vi "Substitute String.vi"(6 "delimeters":cluster{"start":string, "end":string}={"start"="{{", "end"="}}"}, 8 "error in (no error)":errorcluster, 9 "substitutions":map{string, string}(c390), 11 "input string":string) -> (0 "error out":errorcluster, 3 "output string":string)   [LabVIEW 2019]
doc: "<b>Description</b> This VI applies substitutions to the input string using the specified delimeters and substitution lookup table. \n\nFor example, the input string \"{{greeting}}, {{name}}\" would result in the output string \"Hello, World\" if the substituion dictionary contained the mappings {'greeting':'Hello', 'name':'World'}.\n\nThis VI will return an error if the input contains a substitution not found in the dictionary.\n\n\n\n<b>Inputs</b>\n<b>substitutions</b>: A dictoinary of substitutions to apply to the input string.\n<b>delimeters</b>: The start and end delimeters for the desired substitution pattern. Defaults to '{{' and '}}'.\n<b>input string</b>: A string potentially containing substituions.\n\n<b>Outputs</b>\n<b>error out</b>: This VI will return error -1967345147 if a substitution key is missing from the input dictionary.\n<b>output string</b>: A string with substitution keys replaced with values."
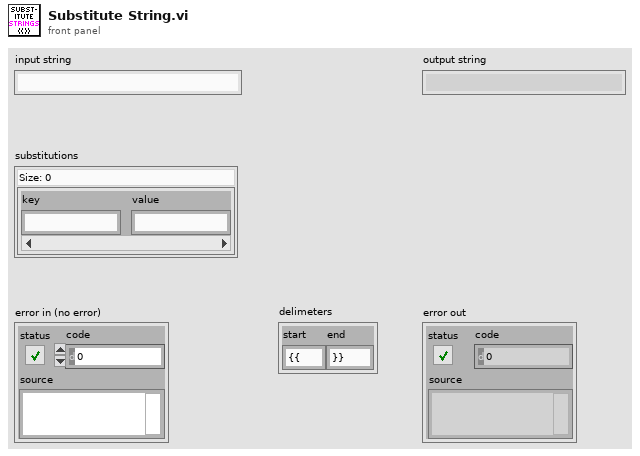
[diagram p1: front panel]
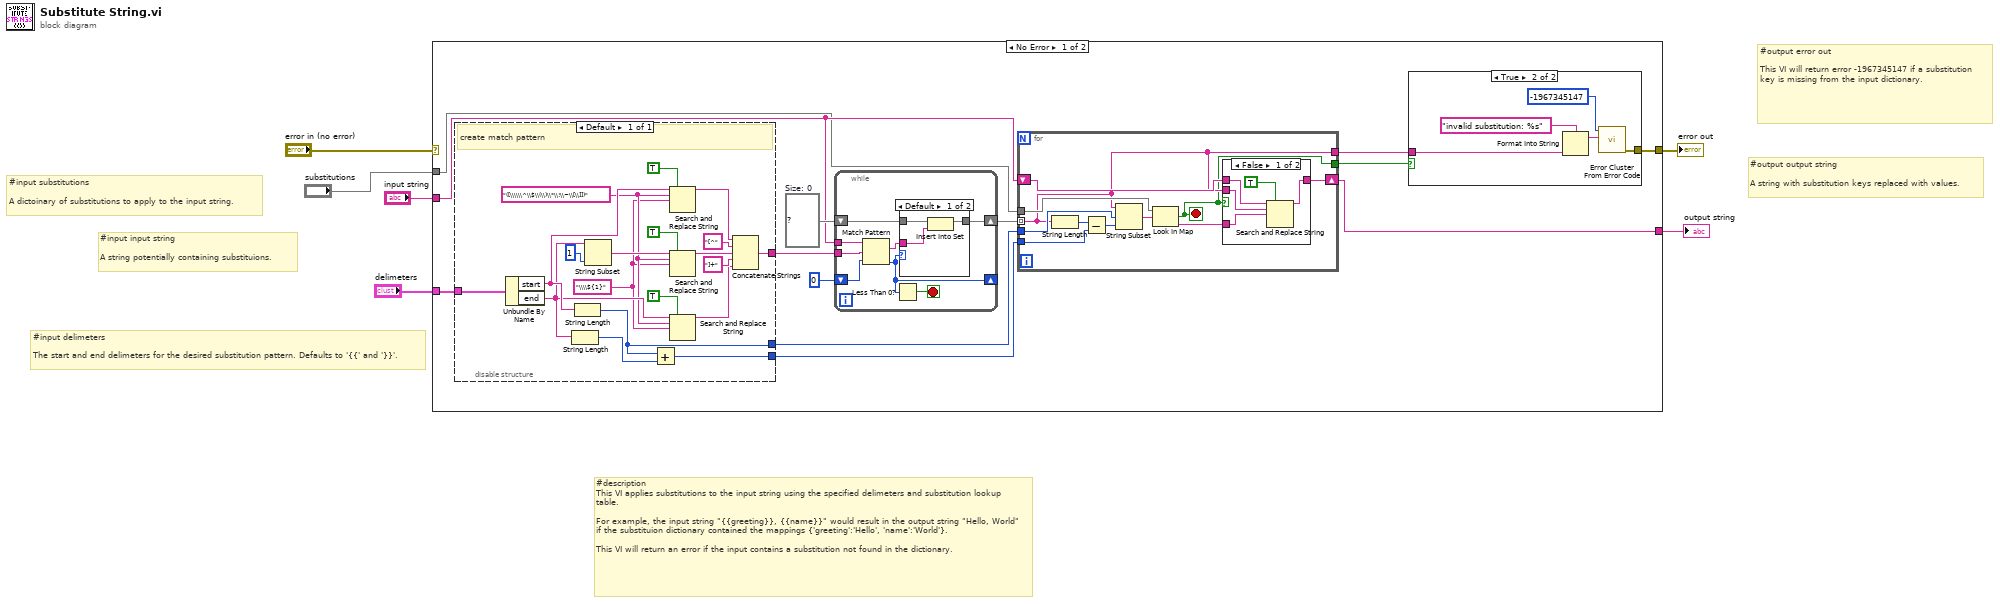
[diagram p0: block diagram]
diagram:
  # "#output error out\n\nThis VI will return error -1967345147 if a substitution key is missing from the input dictionary."
  # "#output output string\n\nA string with substitution keys replaced with values."
  # "#input substitutions\n\nA dictoinary of substitutions to apply to the input string."
  # "#input delimeters\n\nThe start and end delimeters for the desired substitution pattern. Defaults to '{{' and '}}'."
  # "#input input string\n\nA string potentially containing substituions."
  # "#description\nThis VI applies substitutions to the input string using the specified delimeters and substitution lookup table. \n\nFor example, the input string \"{{greeting}}, {{name}}\" would result in the output string \"Hello, World\" if the substituion dictionary contained the mappings {'greeting':'Hello', 'name':'World'}.\n\nThis VI will return an error if the input contains a substitution not found in the dictionary."
  n1 = case shown="No Error" "error in (no error)" {
    selector: "error in (no error)" -> [_ w73]
    tunnel: "delimeters" -> [w19 _]
    tunnel: "input string" -> [w15 _]
    tunnel: "substitutions" -> [w13 _]
    tunnel: [w8 w73] -> w2
    tunnel: [w7 _] -> w1
    frame No Error {
      w17 = set{string} {}  # Size: 0
      n2 = disable-structure shown="Default" {
        disable-tunnel: w19 -> [w60]
        disable-tunnel: [w57] -> w18
        disable-tunnel: [w54] -> w11
        disable-tunnel: [w53] -> w12
        frame Enabled {
          w46 = "\\\\${1}" ("replace string (\"\")")
          w47 = "([\\\\\\^\\$\\(\\)\\*\\!\\~\\[\\]])" ("search string")
          # "create match pattern"
          n3 = Unbundle By Name(w60) -> ("start"=w56:string, "end"=w52:string)
          n4 = String Length(string=w52) -> (length=w55:i32)
          n5 = String Length(string=w56) -> (length=w54:i32)
          n6 = String Subset(string=w52, length (rest)=1 ("length (rest)")) -> (substring=w48:string)  [unwired: 1 in]
          n7 = Add(x=w54, y=w55) -> (x+y=w53:i32)
          n8 = Search and Replace String(replace all?=TRUE ("replace all? (F)"), input string=w56, search string=w47, replace string=w46) -> (result string=w59:string)  [unwired: 4 in, 3 out]
          n9 = Search and Replace String(replace all?=TRUE ("replace all? (F)"), input string=w48, search string=w47, replace string=w46) -> (result string=w44:string)  [unwired: 4 in, 3 out]
          n10 = Search and Replace String(replace all?=TRUE ("replace all? (F)"), input string=w52, search string=w47, replace string=w46) -> (result string=w42:string)  [unwired: 4 in, 3 out]
          n11 = Concatenate Strings(w59, "[^" ("string"), w44, "]+" ("string"), w42) -> (w57:string)
        }
      }
      n12 = while {
        tunnel: w15 -> [w68]
        tunnel: w18 -> [w67]
        shift-right: [w63] -> w14
        shift-left: w17 -> [w64]
        shift-right: [w62] -> _
        shift-left: 0 ("offset past match") -> [w61]
        stop <- w66 stop-if-true
        n13 = Match Pattern(string=w68, regular expression=w67, offset (0)=w61) -> (match substring=w65:string, offset past match=w62:i32)  [unwired: 2 out]
        n14 = Less Than 0?(x=w62) -> (x < 0?=w66:bool)
        n15 = case shown="Default" w62 {
          tunnel: w65 -> [w69 _]
          tunnel: w64 -> [w71 w72]
          tunnel: [w70 w72] -> w63
          frame Default {
            n16 = Insert Into Set(10:w69, 11:w71) -> (3:w70:set{string})  [unwired: 1 out]
          }
          frame -1 {
          }
        }
      }
      n17 = for {
        shift-right: [w27] -> w7
        shift-left: w15 -> [w28]
        tunnel: w14 -> [w26] mode=indexing
        tunnel: w13 -> [w31]
        tunnel: w12 -> [w33]
        tunnel: w11 -> [w32]
        tunnel: [w25] -> w10
        tunnel: [w26] -> w9
        stop <- w25 stop-if-true
        n18 = String Length(string=w26) -> (length=w35:i32)
        n19 = Subtract(x=w35, y=w33) -> (x-y=w34:i32)
        n20 = String Subset(string=w26, offset (0)=w32, length (rest)=w34) -> (substring=w30:string)
        n21 = Look In Map(map=w31, key=w30) -> (key not found?=w25:bool, value=w29:string)  [unwired: 1 in]
        n22 = case shown="False" w25 {
          tunnel: w29 -> [w40 _]
          tunnel: w28 -> [w38 w41]
          tunnel: [w37 w41] -> w27
          tunnel: w26 -> [w36 _]
          frame False {
            n23 = Search and Replace String(replace all?=TRUE ("replace all? (F)"), input string=w38, search string=w36, replace string=w40) -> (result string=w37:string)  [unwired: 4 in, 3 out]
          }
          frame True {
          }
        }
      }
      n24 = case shown="True" w10 {
        tunnel: w9 -> [_ w22]
        tunnel: [_ w20] -> w8
        frame False {
        }
        frame True {
          n25 = Format Into String(format string="invalid substitution: %s", w22) -> (resulting string=w21:string)  [unwired: 2 in, 1 out]
          n26 = call <vilib>:"Error Cluster From Error Code.vi"("error message (\"\")"=w21, "error code (0)"=-1967345147) -> ("error out"=w20:errorcluster)  [unwired: 7 in]
        }
      }
    }
    frame Error {
    }
  }
  "error out" <- w2
  "output string" <- w1
